vi "Set_Coordinates.vi"(1 "Longitude":dbl, 2 "Latitude":dbl, 3 "Degrees?":bool, 4 "Path":path) -> (0 "Succes?":bool)   [LabVIEW 2012]
uses:
  <vilib>/Utility/config.llb/Write Key (Double).vi
  VantagePro.dll
  <vilib>/Utility/config.llb/NI_LVConfig.lvlib
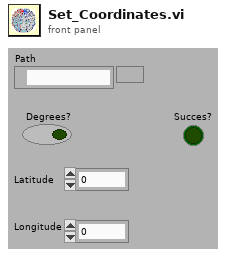
[diagram p1: front panel]
types:
  T1 = typedef "NI_LVConfig.lvlib/Config Data RefNum.ctl" = refnum<k1>
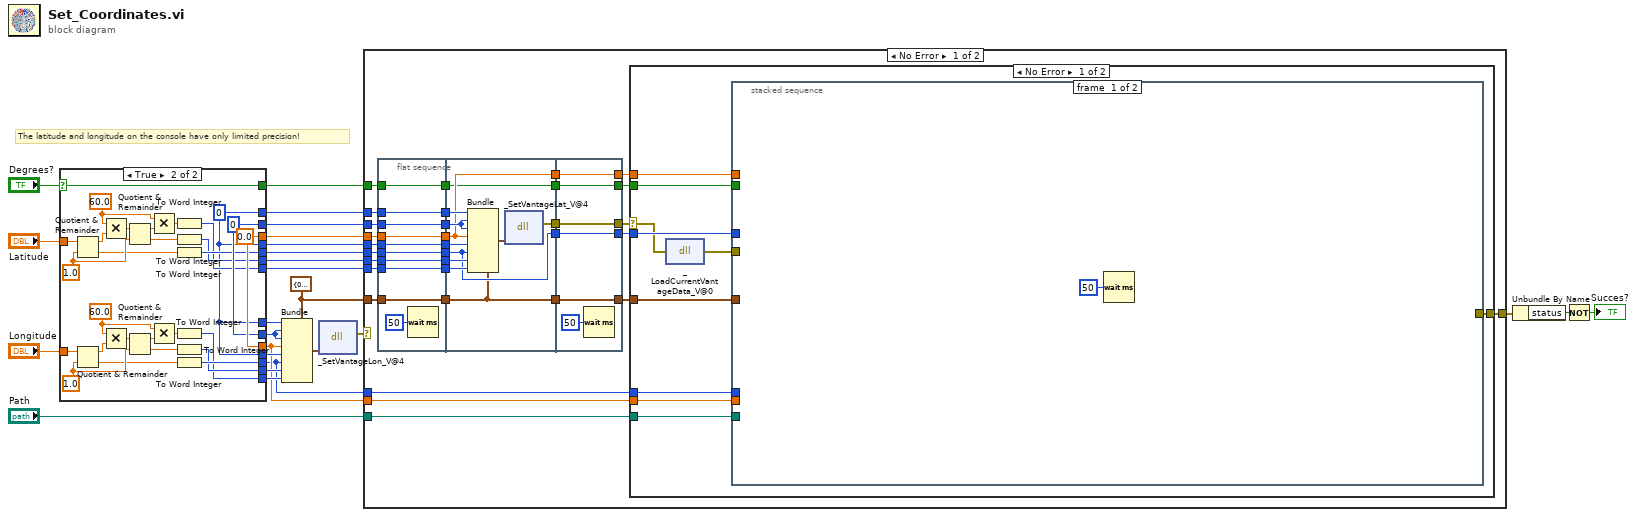
[diagram p0: block diagram]
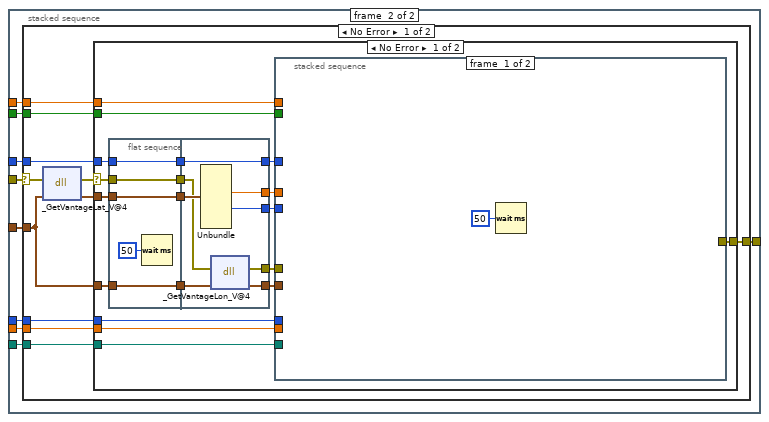
[diagram p2: hidden frame]
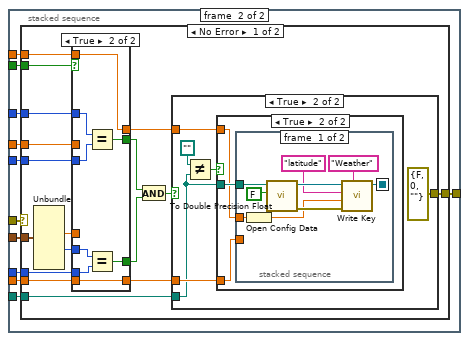
[diagram p3: hidden frame]
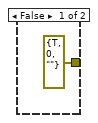
[diagram p4: hidden frame]
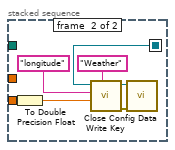
[diagram p6: hidden frame]
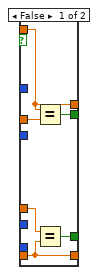
[diagram p7: hidden frame]
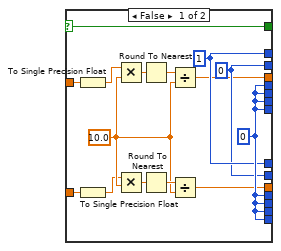
[diagram p13: hidden frame]
diagram:
  w14 = cluster{i16, i8, i8, sgl, i16, i16, i16, i16} {0, 0, 0, 0.0, 0, 0, 0, 0}
  # "The latitude and longitude on the console have only limited precision!"
  n1 = case shown="True" "Degrees?" {
    selector: "Degrees?" -> [w37 w41]
    tunnel: "Latitude" -> [w34 w42]
    tunnel: "Longitude" -> [w29 w43]
    tunnel: [w33 w53] -> w16
    tunnel: [w40 w47] -> w15
    tunnel: [w30 w53] -> w7
    tunnel: [w40 w44] -> w25
    tunnel: [w40 w50] -> w20
    tunnel: [w40 w51] -> w6
    tunnel: [w40 w49] -> w23
    tunnel: [w40 w44] -> w10
    tunnel: [w40 w45] -> w8
    tunnel: [w38 w52] -> w22
    tunnel: [w39 w44] -> w12
    tunnel: [w39 w44] -> w21
    tunnel: [w40 w46] -> w9
    tunnel: [w38 w52] -> w11
    tunnel: [w37 w41] -> w13
    frame False {
      w28 = sgl 10.0 ("y")
      w40 = i16 0
      w39 = i16 1
      w38 = i8 0
      n2 = To Single Precision Float(number=w34) -> (single precision float=w27:sgl)
      n3 = To Single Precision Float(number=w29) -> (single precision float=w26:sgl)
      n4 = Multiply(x=w27, y=w28) -> (x*y=w36:sgl)
      n5 = Multiply(x=w26, y=w28) -> (x*y=w32:sgl)
      n6 = Round To Nearest(number=w36) -> (nearest integer value=w35:sgl)
      n7 = Round To Nearest(number=w32) -> (nearest integer value=w31:sgl)
      n8 = Divide(x=w35, y=w28) -> (x/y=w33:sgl)
      n9 = Divide(x=w31, y=w28) -> (x/y=w30:sgl)
    }
    frame True {
      w52 = i8 0
      w53 = sgl 0.0
      w58 = 60.0 ("x")
      w59 = 1.0 ("y")
      w44 = i16 0
      w65 = 60.0 ("x")
      w66 = 1.0 ("y")
      n10 = Quotient & Remainder(x=w42, y=w66) -> (x-y*floor(x/y)=w68:dbl, floor(x/y)=w63:dbl)
      n11 = Quotient & Remainder(x=w43, y=w59) -> (x-y*floor(x/y)=w61:dbl, floor(x/y)=w56:dbl)
      n12 = Multiply(x=w65, y=w68) -> (x*y=w67:dbl)
      n13 = Multiply(x=w58, y=w61) -> (x*y=w60:dbl)
      n14 = Quotient & Remainder(x=w67, y=w66) -> (x-y*floor(x/y)=w64:dbl, floor(x/y)=w48:dbl)
      n15 = Quotient & Remainder(x=w60, y=w59) -> (x-y*floor(x/y)=w57:dbl, floor(x/y)=w55:dbl)
      n16 = Multiply(x=w65, y=w64) -> (x*y=w62:dbl)
      n17 = Multiply(x=w58, y=w57) -> (x*y=w54:dbl)
      n18 = To Word Integer(number=w62) -> (16bit integer=w45:i16)
      n19 = To Word Integer(number=w48) -> (16bit integer=w46:i16)
      n20 = To Word Integer(number=w63) -> (16bit integer=w47:i16)
      n21 = To Word Integer(number=w54) -> (16bit integer=w49:i16)
      n22 = To Word Integer(number=w55) -> (16bit integer=w50:i16)
      n23 = To Word Integer(number=w56) -> (16bit integer=w51:i16)
    }
  }
  n24 = Bundle(cluster=w14, w21, w22, w22, w7, w25, w6, w20, w23) -> (w5:cluster{i16, i8, i8, sgl, i16, i16, i16, i16})
  n25 = dll-call lib="C:/Users/Bob van Eijk/Desktop/LabView Projects 12/HiSPARC Weather Station/Develop/VantagePro.dll" fn="_SetVantageLon_V@4"("longitude"=w5) -> (error out=w4:errorcluster)  [unwired: 5 in, 1 out]
  n26 = case shown="No Error" w4 {
    selector: w4 -> [_ w264]
    tunnel: [w100 w264] -> w2
    tunnel: "Path" -> [w99 _]
    tunnel: w16 -> [w98 _]
    tunnel: w15 -> [w81 _]
    tunnel: w14 -> [w97 _]
    tunnel: w13 -> [w77 _]
    tunnel: w12 -> [w96 _]
    tunnel: w11 -> [w95 _]
    tunnel: w10 -> [w94 _]
    tunnel: w9 -> [w93 _]
    tunnel: w8 -> [w92 _]
    tunnel: w7 -> [w91 _]
    tunnel: w6 -> [w90 _]
    frame No Error {
      n27 = flat-sequence {
        tunnel: w92 -> [w104]
        tunnel: w93 -> [w105]
        tunnel: w94 -> [w106]
        tunnel: w95 -> [w107]
        tunnel: w96 -> [w108]
        tunnel: w97 -> [w109]
        tunnel: w81 -> [w103]
        tunnel: w98 -> [w110]
        tunnel: [w110] -> w89
        tunnel: [w103] -> w88
        tunnel: [w109] -> w87
        tunnel: [w108] -> w86
        tunnel: [w107] -> w85
        tunnel: [w106] -> w84
        tunnel: [w105] -> w83
        tunnel: [w104] -> w82
        tunnel: w77 -> [w101]
        tunnel: [w101] -> w75
        tunnel: w89 -> [w114]
        tunnel: w88 -> [w115]
        tunnel: w87 -> [w113]
        tunnel: w86 -> [w121]
        tunnel: w85 -> [w120]
        tunnel: w84 -> [w119]
        tunnel: w83 -> [w118]
        tunnel: w82 -> [w117]
        tunnel: w75 -> [w112]
        tunnel: [w115] -> w74
        tunnel: [w114] -> w73
        tunnel: [w113] -> w72
        tunnel: [w112] -> w71
        tunnel: [w111] -> w70
        tunnel: [w124] -> w76
        tunnel: [w125] -> w78
        tunnel: [w126] -> w79
        tunnel: [w127] -> w80
        tunnel: w74 -> [w127]
        tunnel: w73 -> [w126]
        tunnel: w72 -> [w125]
        tunnel: w71 -> [w124]
        tunnel: [w122] -> w69
        tunnel: w70 -> [w122]
        frame #0 {
          n28 = Wait (ms)(milliseconds to wait=u32 50) -> ()  [unwired: 1 out]
        }
        frame #1 {
          n29 = Bundle(cluster=w113, w121, w120, w120, w114, w119, w115, w118, w117) -> (w116:cluster{i16, i8, i8, sgl, i16, i16, i16, i16})
          n30 = dll-call lib="C:/Users/Bob van Eijk/Desktop/LabView Projects 12/HiSPARC Weather Station/Develop/VantagePro.dll" fn="_SetVantageLat_V@4"("latitude"=w116) -> (error out=w111:errorcluster)  [unwired: 5 in, 1 out]
        }
        frame #2 {
          n31 = Wait (ms)(milliseconds to wait=u32 50) -> ()  [unwired: 1 out]
        }
      }
      n32 = case shown="No Error" w69 {
        selector: w69 -> [w129 w263]
        tunnel: [w137 w263] -> w100
        tunnel: w99 -> [w136 _]
        tunnel: w79 -> [w135 _]
        tunnel: w80 -> [w134 _]
        tunnel: w78 -> [w133 _]
        tunnel: w76 -> [w132 _]
        tunnel: w91 -> [w131 _]
        tunnel: w90 -> [w130 _]
        frame No Error {
          n33 = dll-call lib="C:/Users/Bob van Eijk/Desktop/LabView Projects 12/HiSPARC Weather Station/Develop/VantagePro.dll" fn="_LoadCurrentVantageData_V@0" label="Load Current Data"(error in=w129) -> (error out=w128:errorcluster)  [unwired: 3 in, 1 out]
          n34 = stacked-sequence {
            tunnel: [_ w147] -> w137
            tunnel: w136 -> [_ w146]
            tunnel: w135 -> [_ w145]
            tunnel: w134 -> [_ w144]
            tunnel: w133 -> [_ w143]
            tunnel: w132 -> [_ w142]
            tunnel: w131 -> [_ w141]
            tunnel: w130 -> [_ w140]
            tunnel: w128 -> [_ w139]
            frame #0 {
              n35 = Wait (ms)(milliseconds to wait=u32 50) -> ()  [unwired: 1 out]
            }
            frame #1 {
              n36 = case shown="No Error" w139 {
                selector: w139 -> [w149 w262]
                tunnel: w143 -> [w153 _]
                tunnel: [w158 w262] -> w147
                tunnel: w142 -> [w155 _]
                tunnel: w145 -> [w156 _]
                tunnel: w141 -> [w152 _]
                tunnel: w144 -> [w154 _]
                tunnel: w140 -> [w151 _]
                tunnel: w146 -> [w157 _]
                frame No Error {
                  n37 = dll-call lib="C:/Users/Bob van Eijk/Desktop/LabView Projects 12/HiSPARC Weather Station/Develop/VantagePro.dll" fn="_GetVantageLat_V@4" label="Get latitude"(error in=w149, "latitude"=w153) -> (error out=w148:errorcluster, "latitude"=w150:cluster{i16, i8, i8, sgl, i16, i16, i16, i16})  [unwired: 3 in, 1 out]
                  n38 = case shown="No Error" w148 {
                    selector: w148 -> [w166 w261]
                    tunnel: [w175 w261] -> w158
                    tunnel: w157 -> [w174 _]
                    tunnel: w156 -> [w173 _]
                    tunnel: w155 -> [w172 _]
                    tunnel: w154 -> [w162 _]
                    tunnel: w153 -> [w171 _]
                    tunnel: w152 -> [w170 _]
                    tunnel: w151 -> [w169 _]
                    tunnel: w150 -> [w168 _]
                    frame No Error {
                      n39 = flat-sequence {
                        tunnel: w166 -> [w250]
                        tunnel: w168 -> [w251]
                        tunnel: w171 -> [w252]
                        tunnel: [w252] -> w165
                        tunnel: [w251] -> w164
                        tunnel: [w250] -> w163
                        tunnel: w162 -> [w248]
                        tunnel: [w248] -> w160
                        tunnel: [w260] -> w177
                        tunnel: [w259] -> w176
                        tunnel: [w256] -> w167
                        tunnel: w165 -> [w258]
                        tunnel: w164 -> [w257]
                        tunnel: w163 -> [w255]
                        tunnel: [w254] -> w161
                        tunnel: w160 -> [w254]
                        tunnel: [w253] -> w159
                        frame #0 {
                          n40 = Wait (ms)(milliseconds to wait=u32 50) -> ()  [unwired: 1 out]
                        }
                        frame #1 {
                          n41 = Unbundle(w257) -> (w260:sgl, w259:i16)  [unwired: 6 out]
                          n42 = dll-call lib="C:/Users/Bob van Eijk/Desktop/LabView Projects 12/HiSPARC Weather Station/Develop/VantagePro.dll" fn="_GetVantageLon_V@4" label="Get longitude"(error in=w255, w258) -> (error out=w253:errorcluster, w256:cluster{i16, i8, i8, sgl, i16, i16, i16, i16})  [unwired: 3 in, 1 out]
                        }
                      }
                      n43 = stacked-sequence {
                        tunnel: w177 -> [_ w189]
                        tunnel: w176 -> [_ w188]
                        tunnel: [_ w187] -> w175
                        tunnel: w174 -> [_ w186]
                        tunnel: w173 -> [_ w185]
                        tunnel: w172 -> [_ w184]
                        tunnel: w170 -> [_ w183]
                        tunnel: w169 -> [_ w182]
                        tunnel: w167 -> [_ w181]
                        tunnel: w161 -> [_ w180]
                        tunnel: w159 -> [_ w179]
                        frame #0 {
                          n44 = Wait (ms)(milliseconds to wait=u32 50) -> ()  [unwired: 1 out]
                        }
                        frame #1 {
                          n45 = case shown="No Error" w179 {
                            selector: w179 -> [_ w247]
                            tunnel: w189 -> [w206 _]
                            tunnel: w188 -> [w205 _]
                            tunnel: [w190 w247] -> w187
                            tunnel: w186 -> [w202 _]
                            tunnel: w185 -> [w201 _]
                            tunnel: w184 -> [w200 _]
                            tunnel: w183 -> [w199 _]
                            tunnel: w182 -> [w197 _]
                            tunnel: w181 -> [w195 _]
                            tunnel: w180 -> [w194 _]
                            frame No Error {
                              n46 = Unbundle(w195) -> (w198:sgl, w196:i16)  [unwired: 6 out]
                              n47 = case shown="True" w200 {
                                tunnel: [w237 w245] -> w193
                                tunnel: w198 -> [w238 _]
                                tunnel: w206 -> [w236 _]
                                tunnel: w201 -> [w233 w240]
                                tunnel: w199 -> [w234 w239]
                                tunnel: [w235 w246] -> w192
                                tunnel: w194 -> [_ w241]
                                tunnel: w197 -> [_ w244]
                                tunnel: w205 -> [_ w242]
                                tunnel: w196 -> [_ w243]
                                tunnel: [w234 w239] -> w204
                                tunnel: [w233 w240] -> w203
                                frame False {
                                n48 = Equal?(x=w233, y=w236) -> (x = y?=w235:bool)
                                n49 = Equal?(x=w238, y=w234) -> (x = y?=w237:bool)
                                }
                                frame True {
                                n50 = Equal?(x=w241, y=w242) -> (x = y?=w246:bool)
                                n51 = Equal?(x=w243, y=w244) -> (x = y?=w245:bool)
                                }
                              }
                              n52 = And(x=w192, y=w193) -> (x .and. y?=w191:bool)
                              n53 = case shown="True" w191 {
                                tunnel: w204 -> [_ w213]
                                tunnel: w203 -> [_ w212]
                                tunnel: w202 -> [_ w210]
                                tunnel: [errorcluster {"status"=TRUE, "code"=0, "source"=""} ("error IO") errorcluster {"status"=FALSE, "code"=0, "source"=""} ("error IO")] -> w190
                                frame False {
                                }
                                frame True {
                                n54 = Not Equal?(x=path "", y=w210) -> (x != y?=w211:bool)
                                n55 = case shown="True" w211 {
                                tunnel: w210 -> [_ w216]
                                tunnel: w213 -> [_ w215]
                                tunnel: w212 -> [_ w214]
                                frame False {
                                }
                                frame True {
                                n56 = stacked-sequence {
                                seq-local: [w222 _] -> [_ w232]
                                tunnel: w216 -> [w223 _]
                                tunnel: w214 -> [w218 _]
                                tunnel: w215 -> [_ w227]
                                frame #0 {
                                n57 = To Double Precision Float(number=w218) -> (double precision float=w217:dbl)
                                n58 = call <vilib>:"Open Config Data.vi"("create file if necessary (T)"=FALSE, "configuration file path"=w223) -> ("error out"=w219:errorcluster, "refnum"=w224:T1)  [unwired: 7 in, 1 out]
                                n59 = call-poly <vilib>:"Write Key.vi"("section"="Weather" ("key"), "error in (no error)"=w219, "value"=w217, "key"="latitude", "refnum"=w224) -> ("refnum out"=w222:T1)  [unwired: 4 in, 2 out]
                                }
                                frame #1 {
                                n60 = To Double Precision Float(number=w227) -> (double precision float=w226:dbl)
                                n61 = call-poly <vilib>:"Write Key.vi"("section"="Weather" ("key"), "value"=w226, "key"="longitude", "refnum"=w232) -> ("error out"=w228:errorcluster, "refnum out"=w229:T1)  [unwired: 5 in, 1 out]
                                n62 = call <vilib>:"Close Config Data.vi"("error in (no error)"=w228, "refnum"=w229) -> ()  [unwired: 8 in, 2 out]
                                }
                                }
                                }
                                }
                                }
                              }
                            }
                            frame Error {
                            }
                          }
                        }
                      }
                    }
                    frame Error {
                    }
                  }
                }
                frame Error {
                }
              }
            }
          }
        }
        frame Error {
        }
      }
    }
    frame Error {
    }
  }
  n63 = Unbundle By Name(w2) -> ("status"=w3:bool)
  n64 = Not(x=w3) -> (.not. x?=→"Succes?":bool)
